vi "test enum to string to enum.vi"(8 "error in (no error)":errorcluster) -> (0 "error out":errorcluster)   [LabVIEW 2019]
uses:
  lvsrc/Framework/Instrument/Typedefs/Instrument.Commands--Enum.ctl
  8d9037bb-3c7b-4ed9-bda7-cfbc15db33f4.vi
  c1111452-3691-4997-8ea0-ca2c51db40a9.vi
  c1111452-3691-4997-8ea0-ca2c51db40a9.vi/a6fbd7c8-b6df-493a-927f-10650d4a3cdc.vi
  <vilib>/Utility/Data Type/Get Numeric Information.vi
  <vilib>/addons/_JKI Toolkits/Caraya/classes/Assert/Assert Equal Value_Variant.vi
  lvsrc/Framework/Instrument/Instrument.lvclass
  <vilib>/addons/_JKI Toolkits/Caraya/classes/Assert/Assert.lvclass
  <vilib>/addons/_JKI Toolkits/Caraya/classes/Test/Test.lvclass
panel:
  in  "enum in":T1=enum."HELP"
  out "enum out":T1
  out "string out":string
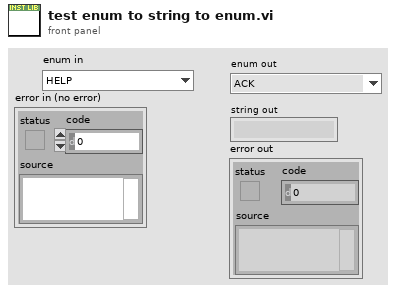
[diagram p1: front panel]
types:
  T1 = typedef "Instrument.lvclass/Instrument.Commands--Enum.ctl" = enum16{"ACK", "HELP", "setConfiguration", "setLogData", "getAll", "getAllData"}
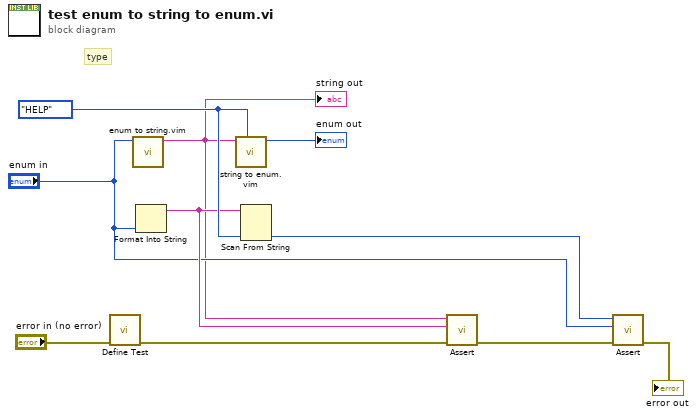
[diagram p0: block diagram]
diagram:
  w9 = Instrument.Commands--Enum."HELP" ("Commands")
  # "type"
  n1 = call <vilib>:"Define Test.vi"("error in (no error)"="error in (no error)") -> ("error out"=w4:errorcluster)  [unwired: 9 in, 1 out]
  n2 = call "enum to string.vim"("enum in"="enum in") -> ("string out"=w3:string)  [unwired: 9 in, 1 out]
  "string out" <- w3
  n3 = Format Into String("enum in") -> (resulting string=w8:string)  [unwired: 3 in, 1 out]
  n4 = call "string to enum.vim"("enum type"=w9, "string in"=w3) -> ("enum out"=→"enum out":T1)  [unwired: 9 in]
  n5 = Scan From String(input string=w8, default 1=w9) -> (output 1=w7:T1)  [unwired: 3 in, 3 out]
  n6 = call-poly <vilib>:"Assert.vi"("error in (no error)"=w4, "Y"=w8, "X"=w3) -> ("error out"=w5:errorcluster)  [unwired: 7 in, 1 out]
  n7 = call-poly <vilib>:"Assert.vi"("error in (no error)"=w5, "Y"="enum in", "X"=w7) -> ("error out"=→"error out":errorcluster)  [unwired: 7 in, 1 out]
